vi "DDE Client Example.vi"() -> ()   [LabVIEW 2015]
panel:
  in  "stop":bool
  out "data":string
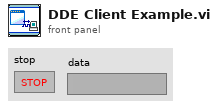
[diagram p1: front panel]
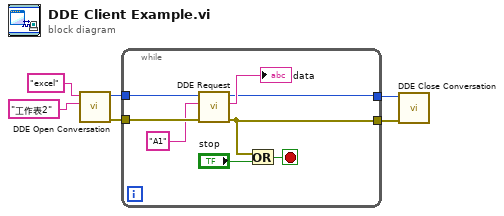
[diagram p0: block diagram]
diagram:
  n1 = call "DDE Open Conversation.vi"("topic"="工作表2" ("service"), "service"="excel" ("topic")) -> ("error out"=w5:errorcluster, "conversation refnum"=w6:u32)  [unwired: 6 in]
  n2 = while {
    tunnel: w6 -> [w14]
    tunnel: w5 -> [w13]
    tunnel: [w10] -> w4
    tunnel: [w9] -> w3
    stop <- w8 stop-if-true
    n3 = call "DDE Request.vi"("error in (no error)"=w13, "item"="A1", "conversation refnum in"=w14) -> ("error out"=w9:errorcluster, "data"=→"data":string, "conversation refnum out"=w10:u32)  [unwired: 4 in]
    n4 = Or(x=w9, y="stop") -> (x .or. y?=w8:bool)
  }
  n5 = call "DDE Close Conversation.vi"("error in (no error)"=w3, "conversation refnum"=w4) -> ()  [unwired: 7 in, 1 out]
